vi "Create.vi"(5 "Comment":refnum<vi>, 7 "Console":refnum<vi>, 8 "error in":errorcluster) -> (0 "error out":errorcluster, 3 "Console Log out":refnum<class "Console Log.lvclass">)   [LabVIEW 2011, in "Console Log.lvclass"]
uses:
  Console Log.lvclass
  Console Log.lvclass/Console Log.ctl
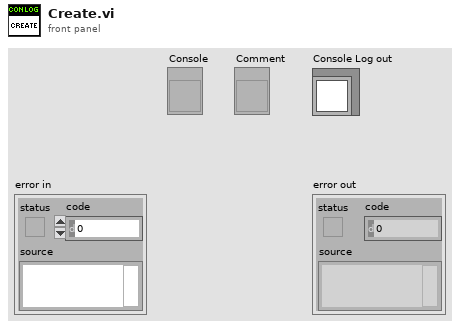
[diagram p1: front panel]
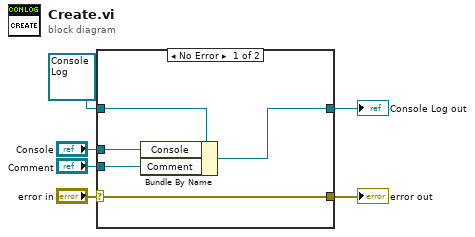
[diagram p0: block diagram]
diagram:
  n1 = case shown="No Error" "error in" {
    selector: "error in" -> [w11 w13]
    tunnel: [w11 w13] -> w5
    tunnel: [w9 w12] -> w3
    tunnel: refnum<class "Console Log.lvclass"> refnum ("Console Log in") -> [w10 w12]
    tunnel: "Console" -> [w8 _]
    tunnel: "Comment" -> [w7 _]
    frame No Error {
      n2 = Bundle By Name(cluster=w10, "Console"=w8, "Comment"=w7) -> (w9:refnum<class "Console Log.lvclass">)
    }
    frame Error {
    }
  }
  "error out" <- w5
  "Console Log out" <- w3
